vi "ELVIS III v1.0 AO Build Bank Data.vi"(8 "error in (no error)":errorcluster, 9 "Wait Until Done?":bool, 10 "Channel Bitmask":bool[](array[boolean]), 11 "dbl Scaled Value List in":i32[][](array[numeric])) -> (0 "error out":errorcluster, 1 "Channel Selected?":bool, 3 "Bank Data":T1 caption="DO (N Samples) Configuration")   [LabVIEW 2021]
uses:
  <vilib>/myRIO/Common/Instrument Driver Framework/ELVIS III v1.0/AO Block/typedefs/ELVIS III AO Block Bank Data.ctl
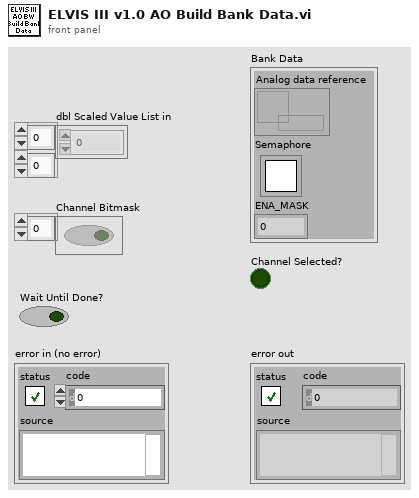
[diagram p1: front panel]
types:
  T1 = typedef "ELVIS III AO Block Bank Data.ctl" = cluster{"Analog data reference":refnum<data-value>, "Semaphore":T2, "ENA_MASK":u8}
  T2 = typedef "Semaphore RefNum" = refnum<k1>
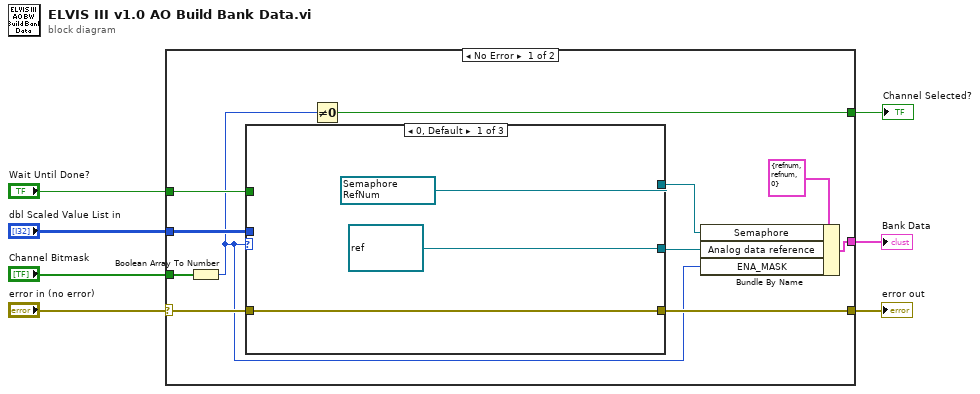
[diagram p0: block diagram]
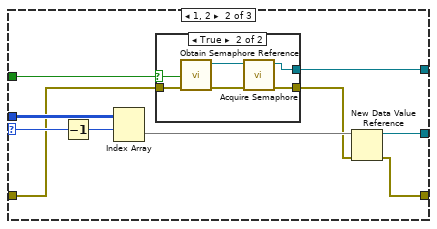
[diagram p2: hidden frame]
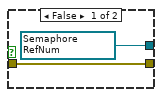
[diagram p3: hidden frame]
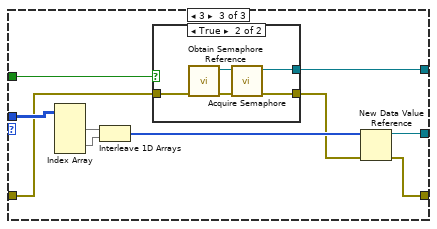
[diagram p4: hidden frame]
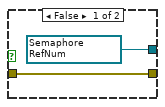
[diagram p5: hidden frame]
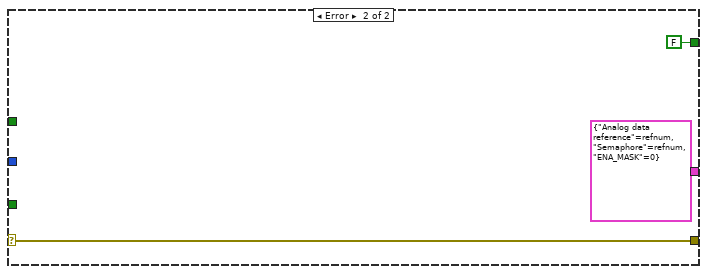
[diagram p6: hidden frame]
diagram:
  n1 = case shown="No Error" "error in (no error)" {
    selector: "error in (no error)" -> [w12 w57]
    tunnel: "Channel Bitmask" -> [w18 _]
    tunnel: [w17 FALSE] -> w6
    tunnel: "Wait Until Done?" -> [w16 _]
    tunnel: [w13 T1 {"Analog data reference"=refnum, "Semaphore"=refnum, "ENA_MASK"=0} ("AO (N Samples) Bank Configuration")] -> w4
    tunnel: [w11 w57] -> w2
    tunnel: "dbl Scaled Value List in" -> [w10 _]
    frame No Error {
      n2 = Boolean Array To Number(Boolean array=w18) -> (number=w9:u8)
      n3 = case shown="0, Default" w9 {
        selector: w9 -> [_ w27 _]
        tunnel: w10 -> [_ w28 w47]
        tunnel: [refnum<data-value> refnum ("Analog data reference") w31 w40] -> w14
        tunnel: w16 -> [_ w30 w49]
        tunnel: w12 -> [w21 w23 w42]
        tunnel: [w21 w29 w48] -> w11
        tunnel: [w20 w24 w43] -> w8
        frame 0, Default {
          w20 = T2 refnum items=["semaphore"] ("semaphore")
        }
        frame 1, 2 {
          n4 = Decrement(x=w27) -> (x-1=w26:u8)
          n5 = Index Array(array=w28, index (row)=w26) -> (element=w25:i32[])  [unwired: 1 in]
          n6 = case shown="True" w30 {
            selector: w30 -> [_ w39]
            tunnel: [w33 w35] -> w24
            tunnel: w23 -> [w32 w38]
            tunnel: [w32 w36] -> w22
            frame False {
              w33 = T2 refnum items=["semaphore"] ("semaphore")
            }
            frame True {
              n7 = call <vilib>:"Obtain Semaphore Reference.vi"("error in (no error)"=w38, "create if not found (T)"=w39) -> ("error out"=w37:errorcluster, "semaphore"=w34:T2)  [unwired: 3 in, 1 out]
              n8 = call <vilib>:"Acquire Semaphore.vi"("error in (no error)"=w37, "semaphore"=w34) -> ("error out"=w36:errorcluster, "semaphore out"=w35:T2)  [unwired: 3 in, 1 out]
            }
          }
          n9 = New Data Value Reference(data value=w25, error in=w22) -> (data value reference=w31:refnum<data-value>, error out=w29:errorcluster)
        }
        frame 3 {
          n10 = Index Array(array=w47) -> (element #1=w46:i32[], element #2=w45:i32[])  [unwired: 4 in]
          n11 = Interleave 1D Arrays(w46, w45) -> (w44:i32[])
          n12 = case shown="True" w49 {
            tunnel: [w51 w53] -> w43
            tunnel: w42 -> [w50 w56]
            tunnel: [w50 w54] -> w41
            frame False {
              w51 = T2 refnum items=["semaphore"] ("semaphore")
            }
            frame True {
              n13 = call <vilib>:"Obtain Semaphore Reference.vi"("error in (no error)"=w56) -> ("error out"=w55:errorcluster, "semaphore"=w52:T2)  [unwired: 4 in, 1 out]
              n14 = call <vilib>:"Acquire Semaphore.vi"("error in (no error)"=w55, "semaphore"=w52) -> ("error out"=w54:errorcluster, "semaphore out"=w53:T2)  [unwired: 3 in, 1 out]
            }
          }
          n15 = New Data Value Reference(data value=w44, error in=w41) -> (data value reference=w40:refnum<data-value>, error out=w48:errorcluster)
        }
      }
      n16 = Not Equal To 0?(x=w9) -> (x != 0?=w17:bool)
      n17 = Bundle By Name(cluster=T1 {"Analog data reference"=refnum, "Semaphore"=refnum, "ENA_MASK"=0} ("AO (N Samples) Bank Configuration"), "Semaphore"=w8, "Analog data reference"=w14, "ENA_MASK"=w9) -> (w13:T1)
    }
    frame Error {
    }
  }
  "Channel Selected?" <- w6
  "Bank Data" <- w4
  "error out" <- w2
